vi "fpga_p3.vi"() -> ()   [LabVIEW 2014]
uses:
  Z:/cloud/LabView/roger-i2c/FPGA/Controls/FPGA I2C_Cmd.ctl
  Z:/cloud/LabView/roger-i2c/FPGA/Controls/FPGA_I2C IO Cluster.ctl
  Z:/cloud/LabView/roger-i2c/FPGA/Controls/FPGA I2C_Comm Loop State.ctl
  <vilib>/rvi/Emulation/niFpgaGetClockAttributes.vi
  <vilib>/rvi/Emulation/niFpgaSctlEmulationGetInTimedLoop.vi
  <vilib>/rvi/Emulation/niFpgaEmulationReportErrorSimple.vi
  <vilib>/rvi/eio/common/nirviEmuTemplateMethod_errors.vi
  <vilib>/rvi/interface/RandomDataEmulation/niFpgaRandomDataHandleErrors.vi
  <vilib>/rvi/Emulation/niFpgaCriticalErrorInLSC.vi
  Z:/cloud/LabView/roger-i2c/FPGA/Code/FPGA I2C_Globals.vi
  <vilib>/rvi/Emulation/niFpgaProcessEmulError.vi
  <vilib>/rvi/Emulation/niFpgaEmulationIsFPGAContextNoSignature.vi
  <vilib>/rvi/errors/niFpgaSetErrorForExecOnDevCompSimple.vi
  <vilib>/rvi/eio/common/nirviEmuReportErrorAndStop.vi
  <vilib>/rvi/DataTransferAndStorage/Container/Common/niFpgaContainerGetUniqueNameForEmu.vi
  <vilib>/rvi/FIFO/Fifo_Resource/nirvififoEmulationSetSize.vi
  <vilib>/rvi/FIFO/Fifo_Resource/nirviFifoEmulationQueueMgr.vi
  <instcachedir>/0/nirviFifoEmulationQueueMgr_E5CAEC123FF24DC58D834DCA3CDAA9B5.lvgen/nirviFifoEmulationQueueMgr_E5CAEC123FF24DC58D834DCA3CDAA9B5_002.vi
  <vilib>/rvi/FIFO/Fifo_Resource/nirvififoEmulationDetermineInputValidOut.vi
  <vilib>/rvi/FIFO/Fifo_Resource/nirvififoEmulationCreateLock.vi
  <vilib>/rvi/FIFO/Fifo_Resource/nirvififoEmulationObtainLock.vi
  <vilib>/rvi/FIFO/Fifo_Resource/nirvififoEmulationReleaseLock.vi
  <vilib>/rvi/occurrence/nirviWaitOnOccurrenceBase.vi
  <vilib>/rvi/errors/nirviReportUnexpectedCaseInternalError.vi
  <vilib>/rvi/errors/nirviReportUnexpectedCaseInternalError (U32).vi
  <vilib>/Utility/error.llb/Clear Errors.vi
  <vilib>/eio/EIONode/EIONode.xnode
  <vilib>/rvi/DataTransferAndStorage/Container/XNode/niFpgaContainer.xnode
  <vilib>/rvi/interface/RandomDataEmulation/nirviRandomDataFpgaReadWriteTemplate.vi
  <vilib>/rvi/FIFO/Fifo_Resource/nirvififoEmulationWrite.vi
  <vilib>/rvi/FIFO/Fifo_Resource/nirvififoEmulationRead.vi
panel:
  in  "I2C_Ack Read":bool
  out "I2C_Read Flag":bool
  out "I2C_Read Data":u8
  in  "I2C_Write Data":u8
  in  "I2C_Write Flag":bool
  in  "I2C_Wait Time":u32=400
  in  "I2C_Wait Time/2":u32=200
  in  "I2C_Cmd":T1
  in  "I2C_Port":u8
  in  "I2C_Bytes to Read":u16=1
  in  "I2C_Bytes to Write":u16=1
  in  "I2C_Address":u16
  in  "I2C_Start":bool
  in  "Count(uSec)":u32=10
  out "Current Sensor":fxp<+/-,24,5>
  out "Break Sensor":fxp<+/-,24,5>
  out "Steering Angle":fxp<+/-,24,5>
  out "Suspension R-L":fxp<+/-,24,5>
  out "Suspension F-R":fxp<+/-,24,5>
  out "Suspensione R-R":fxp<+/-,24,5>
  out "Suspensione F-L":fxp<+/-,24,5>
  out "=< Lopp time?":bool
  out "Fifo Overflow?":bool
  out "Loop Time":u32
  in  "stop":bool
  in  "Stop Light":bool
  in  "FPGA LED":bool
  in  "Buzzer":bool
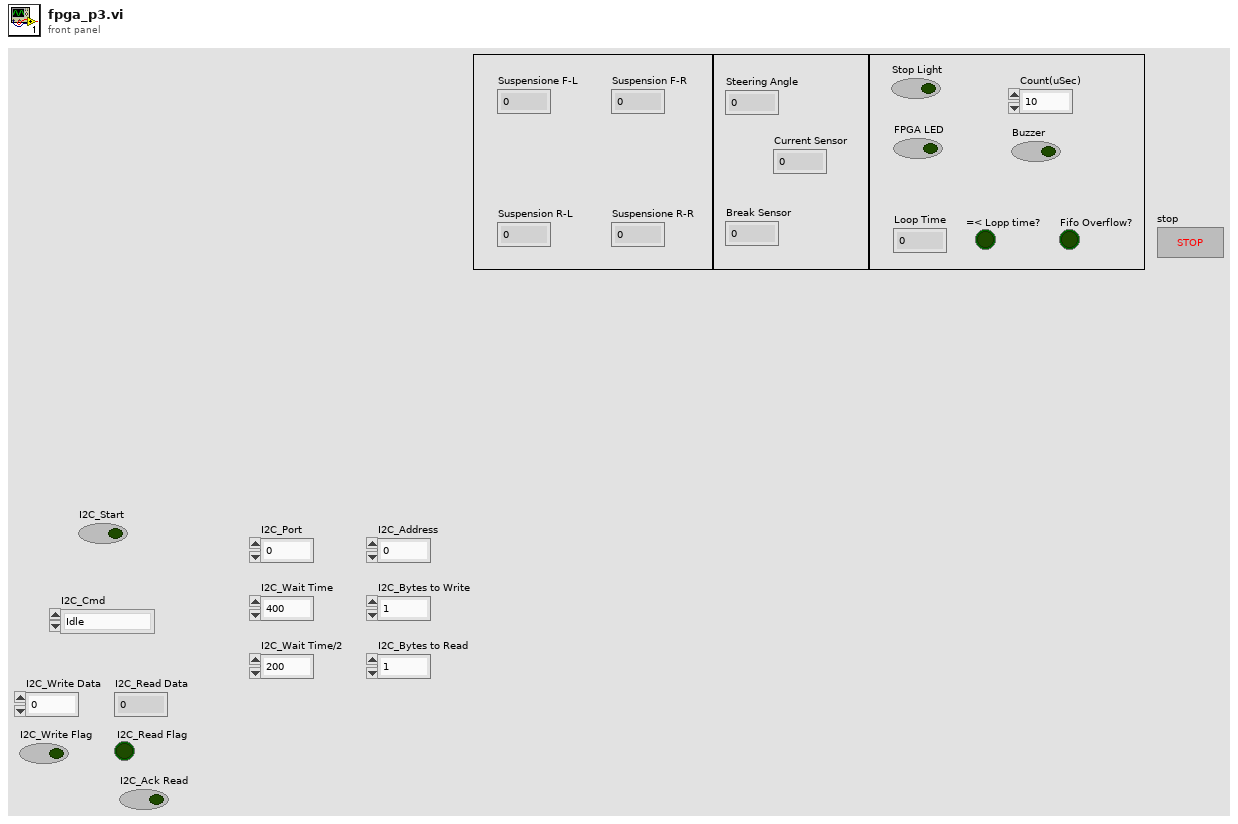
[diagram p1: front panel]
types:
  T1 = typedef "FPGA I2C_Cmd.ctl" = enum8{"Idle", "Write I2C", "Read I2C", "Write & Read I2C", "Configure"}
  T2 = typedef "FPGA I2C_Comm Loop State.ctl" = enum8{"Idle", "Init", "Write", "Start", "Read", "Wait Until Done"}
  T3 = typedef "FPGA_I2C IO Cluster.ctl" = cluster{"SCK":refnum<k21>, "DATA":refnum<k21>}
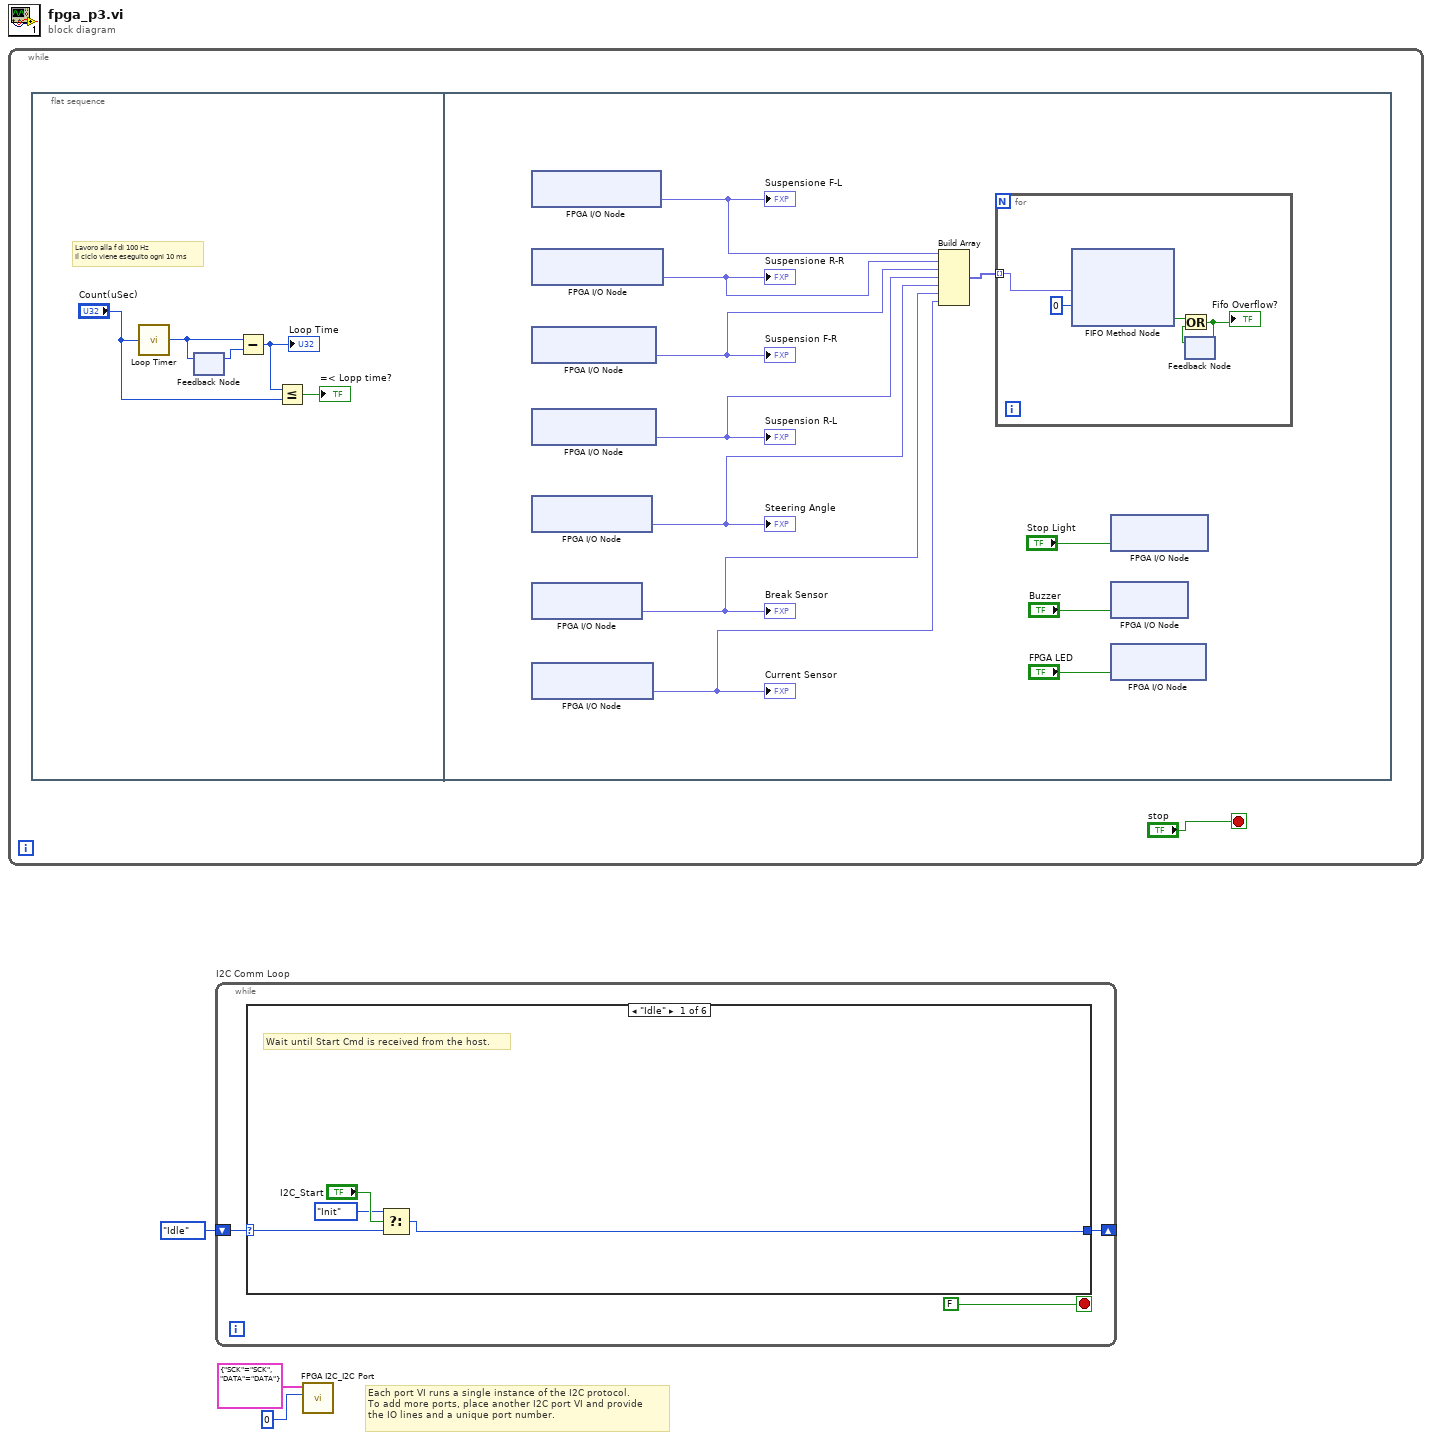
[diagram p0: block diagram]
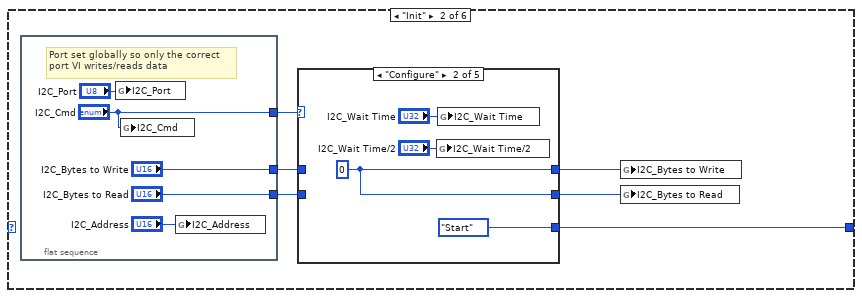
[diagram p2: hidden frame]
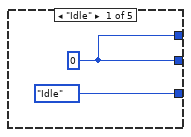
[diagram p3: hidden frame]
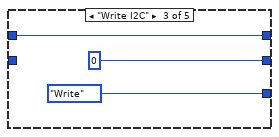
[diagram p4: hidden frame]
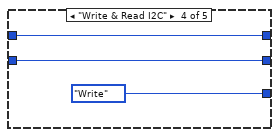
[diagram p5: hidden frame]
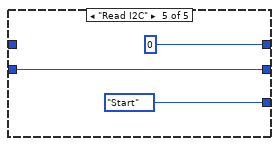
[diagram p6: hidden frame]
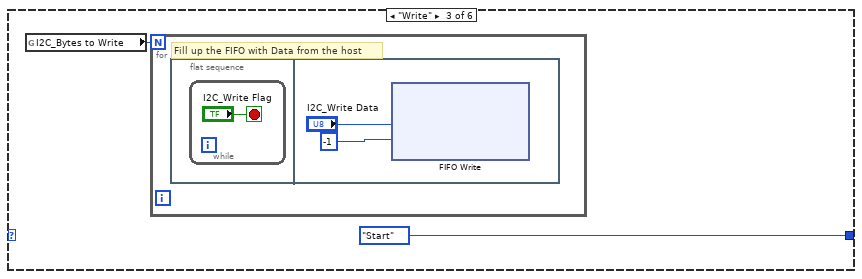
[diagram p7: hidden frame]
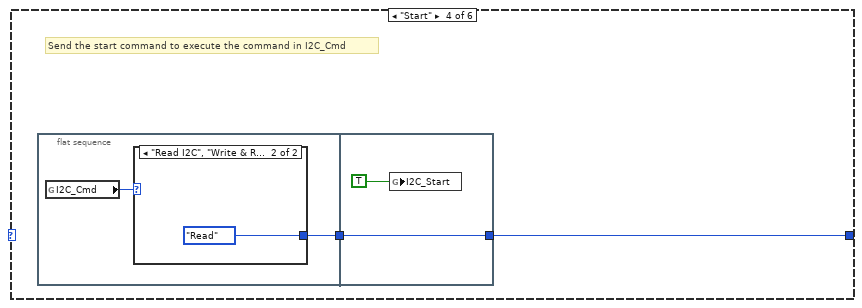
[diagram p8: hidden frame]
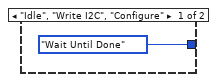
[diagram p9: hidden frame]
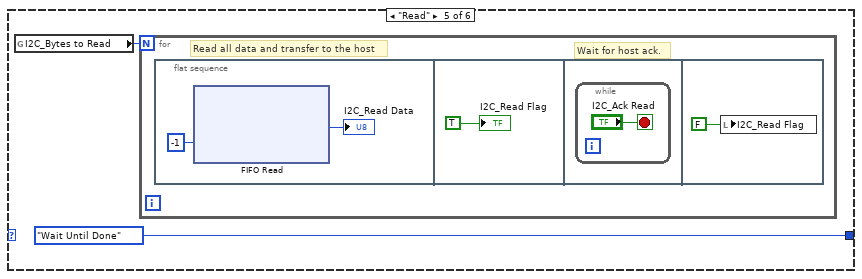
[diagram p10: hidden frame]
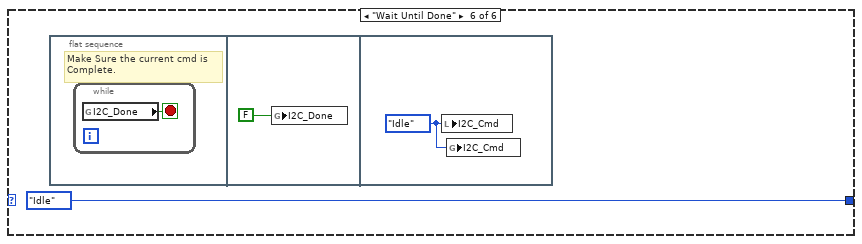
[diagram p11: hidden frame]
diagram:
  # "Each port VI runs a single instance of the I2C protocol.\nTo add more ports, place another I2C port VI and provide\nthe IO lines and a unique port number."
  n1 = while {
    stop <- "stop" stop-if-true
    n2 = flat-sequence {
      frame #0 {
        # "Lavoro alla f di 100 Hz\nIl ciclo viene eseguito ogni 10 ms"
        n3 = call "Loop Timer"("Count(mSec)"="Count(uSec)") -> ("Tick Count(mSec)"=w9:u8)
        n4 = feedback #1() -> (w8:u8)  [unwired: 1 in]
        n5 = feedback-in #1(w9) -> ()
        n6 = Subtract(x=w9, y=w8) -> (x-y=w7:u8)
        "Loop Time" <- w7
        n7 = Less Or Equal?(x=w7, y="Count(uSec)") -> (x <= y?=→"=< Lopp time?":bool)
      }
      frame #1 {
        n8 = xnode "FPGA I/O Node"() -> ("Suspensione F-L"=w16:fxp<+/-,24,5>)  [unwired: 1 in, 1 out]
        "Suspensione F-L" <- w16
        n9 = xnode "FPGA I/O Node"() -> ("Suspensione R-R"=w15:fxp<+/-,24,5>)  [unwired: 1 in, 1 out]
        "Suspensione R-R" <- w15
        n10 = xnode "FPGA I/O Node"() -> ("Suspension F-R"=w14:fxp<+/-,24,5>)  [unwired: 1 in, 1 out]
        "Suspension F-R" <- w14
        n11 = xnode "FPGA I/O Node"() -> ("Suspension R-L"=w13:fxp<+/-,24,5>)  [unwired: 1 in, 1 out]
        "Suspension R-L" <- w13
        n12 = xnode "FPGA I/O Node"() -> ("Steering Angle"=w12:fxp<+/-,24,5>)  [unwired: 1 in, 1 out]
        "Steering Angle" <- w12
        n13 = xnode "FPGA I/O Node"() -> ("Break Sensor"=w11:fxp<+/-,24,5>)  [unwired: 1 in, 1 out]
        "Break Sensor" <- w11
        n14 = xnode "FPGA I/O Node"() -> ("Current Sensor"=w10:fxp<+/-,24,5>)  [unwired: 1 in, 1 out]
        "Current Sensor" <- w10
        n15 = Build Array(w16, w15, w14, w13, w12, w11, w10) -> (w18:fxp<+/-,24,5>[])
        n16 = for {
          tunnel: w18 -> [w21] mode=indexing
          n17 = xnode ("FIFO Method Node")("Element"=w21, "Timeout"=0) -> ("Timed Out?"=w24:bool)  [unwired: 1 in, 1 out]
          n18 = feedback #2() -> (w23:bool)  [unwired: 1 in]
          n19 = Or(x=w24, y=w23) -> (x .or. y?=w22:bool)
          "Fifo Overflow?" <- w22
          n20 = feedback-in #2(w22) -> ()
        }
        n21 = xnode "FPGA I/O Node"("Stop Light"="Stop Light") -> ()  [unwired: 1 in, 1 out]
        n22 = xnode "FPGA I/O Node"("Buzzer"="Buzzer") -> ()  [unwired: 1 in, 1 out]
        n23 = xnode "FPGA I/O Node"("FPGA LED"="FPGA LED") -> ()  [unwired: 1 in, 1 out]
      }
    }
  }
  n24 = while "I2C Comm Loop" {
    shift-right: [w27] -> _
    shift-left: FPGA_I2C_Comm_Loop_State."Idle" ("Action") -> [w26]
    stop <- FALSE stop-if-true
    n25 = case shown="\"Idle\"" w26 {
      selector: w26 -> [w31 _ _ _ _ _]
      tunnel: [w29 w37 FPGA_I2C_Comm_Loop_State."Start" ("Action") w65 FPGA_I2C_Comm_Loop_State."Wait Until Done" ("Action") FPGA_I2C_Comm_Loop_State."Idle" ("Action")] -> w27
      frame "Idle" {
        # "Wait until Start Cmd is received from the host."
        n26 = Select(t=FPGA_I2C_Comm_Loop_State."Init" ("Action"), s="I2C_Start", f=w31) -> (s? t:f=w29:T2)
      }
      frame "Init" {
        n27 = flat-sequence {
          tunnel: ["I2C_Cmd"] -> w38
          tunnel: ["I2C_Bytes to Write"] -> w36
          tunnel: ["I2C_Bytes to Read"] -> w34
          frame #0 {
            # "Port set globally so only the correct\nport VI writes/reads data"
            n28 = global write "FPGA I2C_Globals.vi" "I2C_Port"("I2C_Port") -> ()
            n29 = global write "FPGA I2C_Globals.vi" "I2C_Cmd"("I2C_Cmd") -> ()
            n30 = global write "FPGA I2C_Globals.vi" "I2C_Address"("I2C_Address") -> ()
          }
        }
        n31 = case shown="\"Configure\"" w38 {
          tunnel: [FPGA_I2C_Comm_Loop_State."Idle" ("Action") FPGA_I2C_Comm_Loop_State."Start" ("Action") FPGA_I2C_Comm_Loop_State."Write" ("Action") FPGA_I2C_Comm_Loop_State."Write" ("Action") FPGA_I2C_Comm_Loop_State."Start" ("Action")] -> w37
          tunnel: [w44 w46 w51 w54 u16 0 ("I2C_Bytes to Read")] -> w35
          tunnel: w36 -> [_ _ w51 w54 _]
          tunnel: w34 -> [_ _ _ w53 w56]
          tunnel: [w44 w46 u16 0 ("I2C_Bytes to Read") w53 w56] -> w33
          frame "Idle" {
            w44 = u16 0 ("I2C_Bytes to Read")
          }
          frame "Configure" {
            w46 = u16 0 ("I2C_Bytes to Read")
            n32 = global write "FPGA I2C_Globals.vi" "I2C_Wait Time/2"("I2C_Wait Time/2") -> ()
            n33 = global write "FPGA I2C_Globals.vi" "I2C_Wait Time"("I2C_Wait Time") -> ()
          }
          frame "Write I2C" {
          }
          frame "Write & Read I2C" {
          }
          frame "Read I2C" {
          }
        }
        n34 = global write "FPGA I2C_Globals.vi" "I2C_Bytes to Write"(w35) -> ()
        n35 = global write "FPGA I2C_Globals.vi" "I2C_Bytes to Read"(w33) -> ()
      }
      frame "Write" {
        n36 = global read "FPGA I2C_Globals.vi" "I2C_Bytes to Write"() -> (w59:u16)
        n37 = for {
          N: w59 -> [_]
          # "Fill up the FIFO with Data from the host"
          n38 = flat-sequence {
            frame #0 {
              n39 = while {
                stop <- "I2C_Write Flag" stop-if-true
              }
            }
            frame #1 {
              n40 = xnode ("FIFO Write")("Element"="I2C_Write Data", "Timeout"=-1) -> ()  [unwired: 1 in, 2 out]
            }
          }
        }
      }
      frame "Start" {
        # "Send the start command to execute the command in I2C_Cmd"
        n41 = flat-sequence {
          tunnel: [w67] -> w64
          tunnel: [w71] -> w65
          tunnel: w64 -> [w71]
          frame #0 {
            n42 = global read "FPGA I2C_Globals.vi" "I2C_Cmd"() -> (w66:T1)
            n43 = case shown="\"Read I2C\", \"Write & Read I2C\"" w66 {
              tunnel: [FPGA_I2C_Comm_Loop_State."Wait Until Done" ("Action") FPGA_I2C_Comm_Loop_State."Read" ("Action")] -> w67
              frame "Idle", "Write I2C", "Configure" {
              }
              frame "Read I2C", "Write & Read I2C" {
              }
            }
          }
          frame #1 {
            n44 = global write "FPGA I2C_Globals.vi" "I2C_Start"(TRUE ("Write Flag")) -> ()
          }
        }
      }
      frame "Read" {
        n45 = global read "FPGA I2C_Globals.vi" "I2C_Bytes to Read"() -> (w72:u16)
        n46 = for {
          N: w72 -> [_]
          # "Wait for host ack."
          # "Read all data and transfer to the host"
          n47 = flat-sequence {
            frame #0 {
              n48 = xnode ("FIFO Read")("Timeout"=-1) -> ("Element"=→"I2C_Read Data":u8)  [unwired: 1 in, 2 out]
            }
            frame #1 {
              "I2C_Read Flag" <- TRUE ("Read Flag")
            }
            frame #2 {
              n49 = while {
                stop <- "I2C_Ack Read" stop-if-true
              }
            }
            frame #3 {
              n50 = local write "I2C_Read Flag"(FALSE ("Read Flag")) -> ()
            }
          }
        }
      }
      frame "Wait Until Done" {
        n51 = flat-sequence {
          frame #0 {
            # "Make Sure the current cmd is\nComplete."
            n52 = while {
              stop <- w80 stop-if-true
              n53 = global read "FPGA I2C_Globals.vi" "I2C_Done"() -> (w80:bool)
            }
          }
          frame #1 {
            n54 = global write "FPGA I2C_Globals.vi" "I2C_Done"(FALSE ("Done")) -> ()
          }
          frame #2 {
            w82 = FPGA_I2C_Cmd."Idle" ("I2C_Cmd")
            n55 = local write "I2C_Cmd"(w82) -> ()
            n56 = global write "FPGA I2C_Globals.vi" "I2C_Cmd"(w82) -> ()
          }
        }
      }
    }
  }
  n57 = call "FPGA I2C_I2C Port.vi"("Port"=u8 0, "IO Cluster"=T3 {"SCK"="SCK", "DATA"="DATA"}) -> ()  [unwired: 10 out]
